vi "GT 2D Compare Set Prm.vi"(8 "error in (no error)":errorcluster caption="错误输入（无错误）", 9 "pPrm":T1, 10 "chn":i16, 11 "cardNum":i16) -> (0 "error out":errorcluster caption="错误输出", 1 "pPrm out":T1, 3 "function return":i16)   [LabVIEW 2014, in "gts.lvlib"]
doc: "GT_API GT_2DCompareSetPrm(short cardNum,short chn,T2DComparePrm *pPrm);"
uses:
  gts.lvlib
  gts.dll
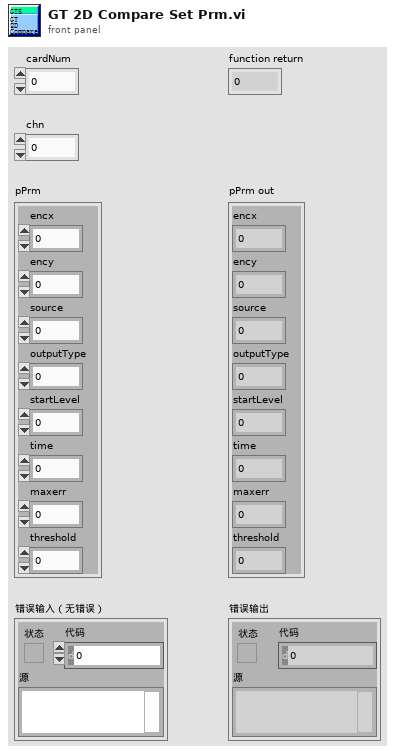
[diagram p1: front panel]
types:
  T1 = cluster{"encx":i16, "ency":i16, "source":i16, "outputType":i16, "startLevel":i16, "time":i16, "maxerr":i16, "threshold":i16}
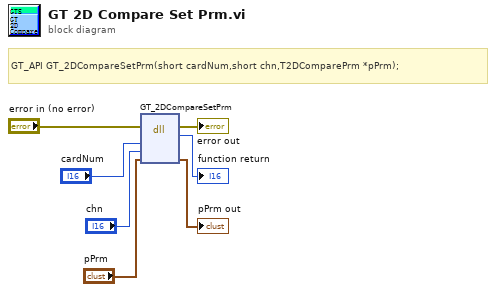
[diagram p0: block diagram]
diagram:
  # "GT_API GT_2DCompareSetPrm(short cardNum,short chn,T2DComparePrm *pPrm);"
  n1 = dll-call lib="PTH2>abs F.多卡库-控制卡基本运动例程(labview)gts.*" fn="GT_2DCompareSetPrm"(error in="error in (no error)", "cardNum"="cardNum", "chn"="chn", "pPrm"="pPrm") -> (error out=→"error out":errorcluster, →"function return":i16, "pPrm"=→"pPrm out":T1)  [unwired: 4 in, 1 out]
